vi "WaypointAndObstaclesPaint 2.vi"(11 "Simulated Initial Robot GPS Info:":dbl[](array[numeric])=[37.1526, 81.2675]) -> (0 "Obs longs":dbl[](array[numeric]) format="%#_8g", 1 "WP Longs":dbl[](array[numeric]) format="%#_8g", 2 "WP Lats":dbl[](array[numeric]) format="%#_8g", 3 "Obs Lats":dbl[](array[numeric]) format="%#_8g")   [LabVIEW 2014]
panel:
  out "480 by 480 array":u8[][](array[numeric])
  # "Waypoint and Obstacles Paint 2"
  # "Inputs:"
  # "Outputs:"
  # "Obstacle latitudes:"
  # "Obstacle Longitudes:"
  # "WP latitudes:"
  # "WP longitudes:"
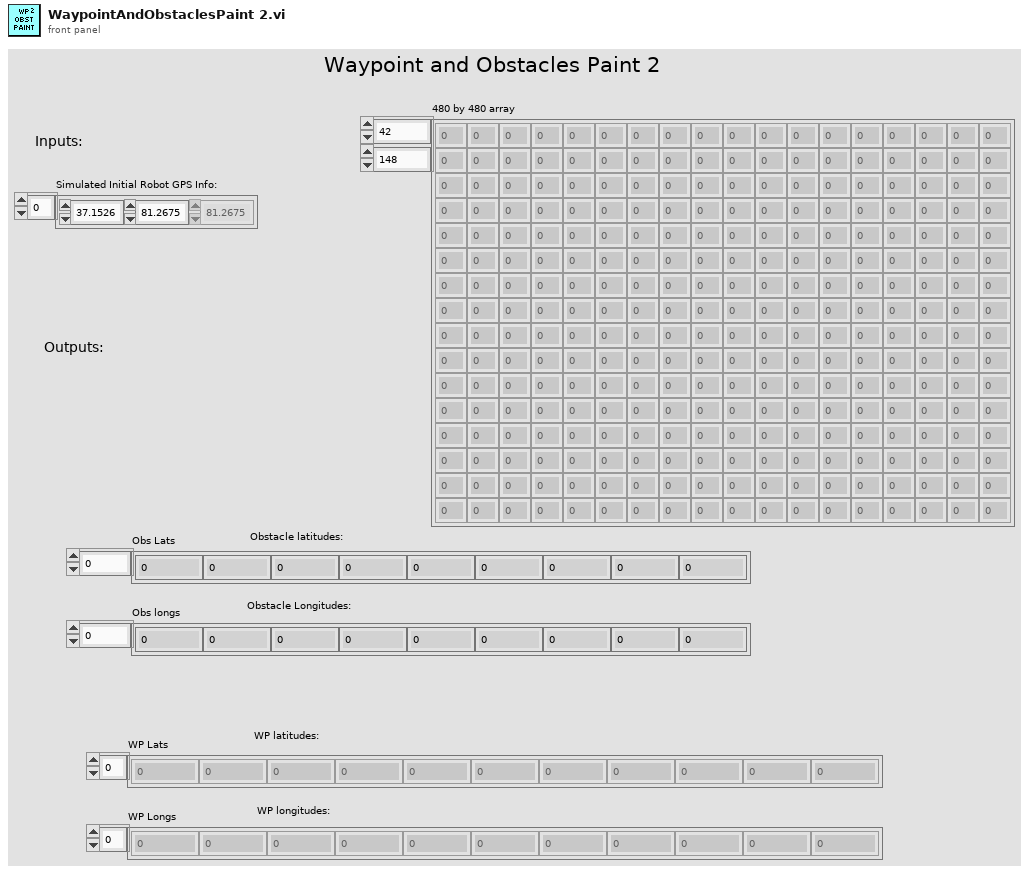
[diagram p1: front panel]
types:
  T1 = typedef "imagedata.ctl" = cluster{"image type":i32, "image depth":i32, "image":u8[], "mask":u8[], "colors":u32[], "Rectangle":cluster{"left":i16, "top":i16, "right":i16, "bottom":i16}}
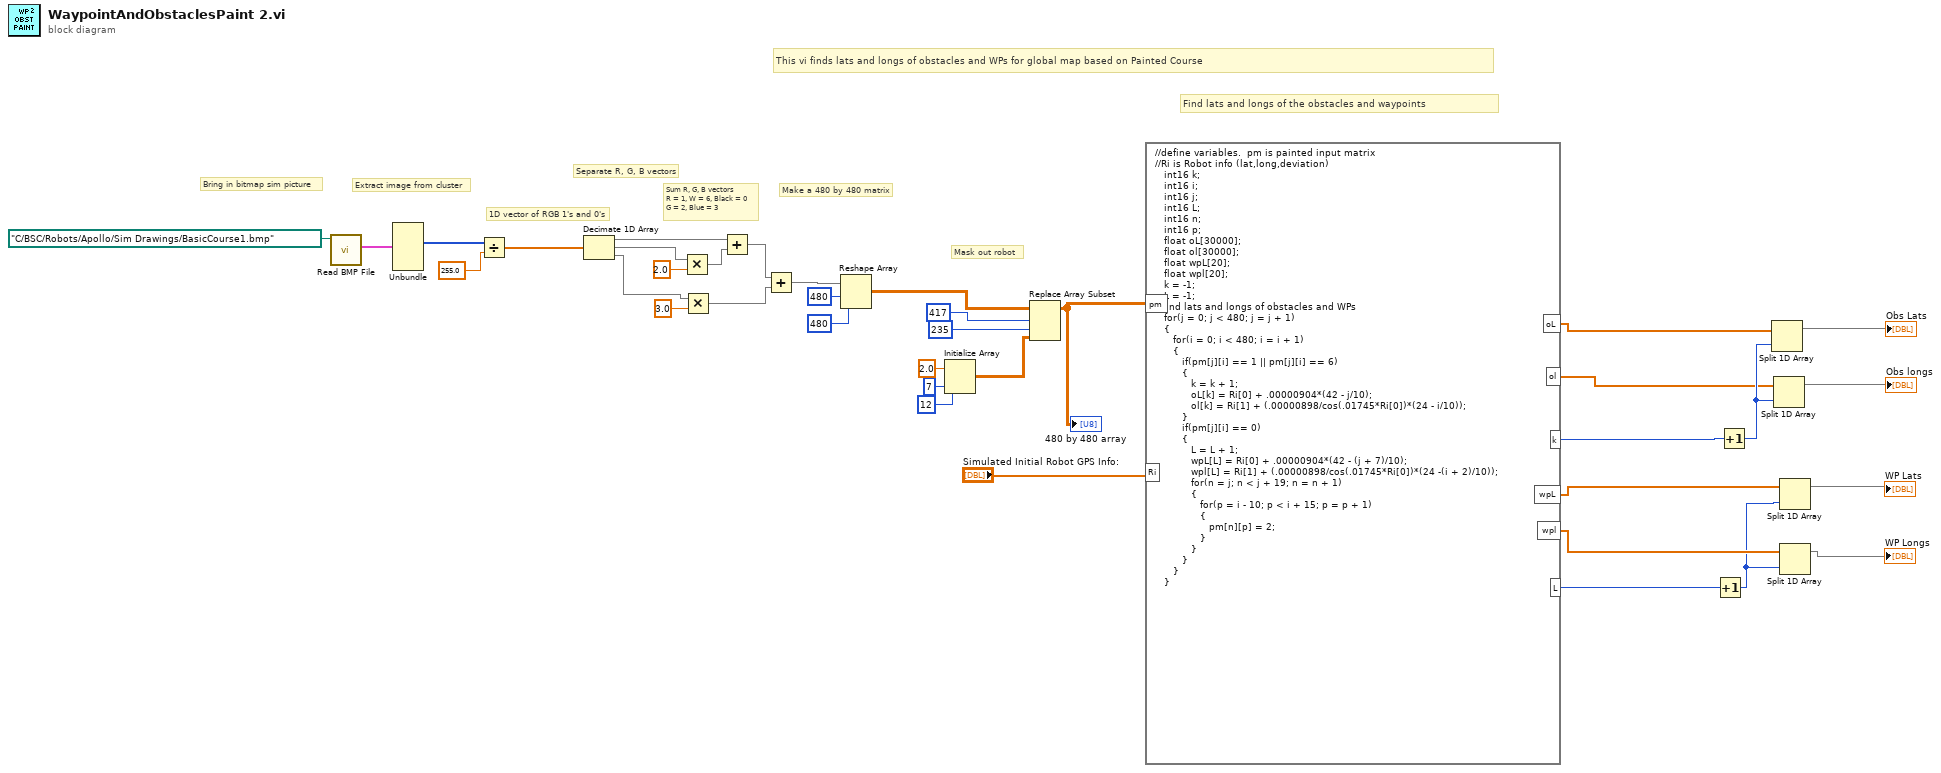
[diagram p0: block diagram]
diagram:
  # "Mask out robot"
  # "Make a 480 by 480 matrix"
  # "Sum R, G, B vectors\nR = 1, W = 6, Black = 0\nG = 2, Blue = 3"
  # "1D vector of RGB 1's and 0's"
  # "This vi finds lats and longs of obstacles and WPs for global map based on Painted Course"
  # "Find lats and longs of the obstacles and waypoints"
  # "Separate R, G, B vectors"
  # "Extract image from cluster"
  # "Bring in bitmap sim picture"
  n1 = call <vilib>:"Read BMP File.vi"("path to BMP file"=path "C:/BSC/Robots/Apollo/Sim Drawings/BasicCourse1.bmp") -> ("image data"=w36:T1)  [unwired: 8 in, 2 out]
  n2 = Unbundle(w36) -> ("image"=w31:u8[])  [unwired: 5 out]
  n3 = Divide(x=w31, y=255.0) -> (x/y=w30:dbl[])
  n4 = Decimate 1D Array(w30) -> (w22:dbl[], w28:dbl[], w26:dbl[])
  n5 = Multiply(x=w28, y=2.0) -> (x*y=w25:dbl[])
  n6 = Multiply(x=w26, y=3.0) -> (x*y=w23:dbl[])
  n7 = Add(x=w22, y=w25) -> (x+y=w24:dbl[])
  n8 = Add(x=w24, y=w23) -> (x+y=w21:dbl[])
  n9 = Reshape Array(w21, 480 ("dimension size"), 480 ("dimension size")) -> (w13:dbl[][])
  n10 = Initialize Array(2.0 ("element"), 7 ("dimension size"), 12 ("dimension size")) -> (w12:dbl[][])
  n11 = Replace Array Subset(array=w13, new element=w12, index (row)=417, index (col)=235) -> (w10:dbl[][])
  "480 by 480 array" <- w10
  n12 = formula code="//define variables.  pm is painted input matrix\n//Ri is Robot info (lat,long,deviation)\n   int16 k;\n   int16 i;\n   int16 j;\n   int16 L;\n   int16 n;\n   int16 p;\n   float oL[30000];\n   float ol[30000];\n   float wpL[20];\n   float wpl[20];\n   k = -1;\n   L = -1;\n//Find lats and longs of obstacles and WPs\n   for(j = 0; j < 480; j = j + 1)\n   {\n      for(i = 0; i < 480; i = i + 1)\n      {\n         if(pm[j][i] == 1 || pm[j][i] == 6)   \n         {\n            k = k + 1;\n            oL[k] = Ri[0] + .00000904*(42 - j/10);\n            ol[k] = Ri[1] + (.00000898/cos(.01745*Ri[0])*(24 - i/10));\n         }\n         if(pm[j][i] == 0)\n         {\n            L = L + 1;\n            wpL[L] = Ri[0] + .00000904*(42 - (j + 7)/10);\n            wpl[L] = Ri[1] + (.00000898/cos(.01745*Ri[0])*(24 -(i + 2)/10));\n            for(n = j; n < j + 19; n = n + 1)\n            {\n               for(p = i - 10; p < i + 15; p = p + 1)\n               {\n                  pm[n][p] = 2;\n               }\n            }\n         }\n      }\n   }"("pm"=w10, "Ri"="Simulated Initial Robot GPS Info:") -> ("oL"=w9:dbl[], "ol"=w8:dbl[], "k"=w7:i16, "wpL"=w6:dbl[], "wpl"=w5:dbl[], "L"=w4:i16)
  n13 = Increment(x=w4) -> (x+1=w3:i16)
  n14 = Increment(x=w7) -> (x+1=w33:i16)
  n15 = Split 1D Array(array=w9, index=w33) -> (first subarray=→"Obs Lats":dbl[])  [unwired: 1 out]
  n16 = Split 1D Array(array=w8, index=w33) -> (first subarray=→"Obs longs":dbl[])  [unwired: 1 out]
  n17 = Split 1D Array(array=w6, index=w3) -> (first subarray=→"WP Lats":dbl[])  [unwired: 1 out]
  n18 = Split 1D Array(array=w5, index=w3) -> (first subarray=→"WP Longs":dbl[])  [unwired: 1 out]
